vi "Get Shutdown Data.vi"(8 "error in (no error)":errorcluster, 10 "Splitter":refnum<vi>, 11 "Message Log in":refnum<class "Message Log.lvclass">) -> (0 "error out":errorcluster, 2 "Data":T1, 3 "Message Log out":refnum<class "Message Log.lvclass">)   [LabVIEW 2017, in "Message Log.lvclass"]
uses:
  Message Log.lvclass
  Config Data.ctl
  <vilib>/Utility/miscctls.llb/LVRectTypeDef.ctl
  C:/Program Files (x86)/National Instruments/LabVIEW 2017/vi.lib/addons/_Workers/Library/Classes/Worker/Worker.lvclass
  Message Log.lvclass/Message Log.ctl
  <vilib>/addons/_Workers/Library/Classes/Worker/Worker.lvclass/Worker.ctl
  <vilib>/Utility/miscctls.llb/LVRowAndColumnTypeDef.ctl
  <vilib>/addons/_Workers/Library/Classes/Worker/Read MainVI Ref DVR.vi
  <vilib>/addons/_Workers/Library/Classes/Worker/Worker.lvclass
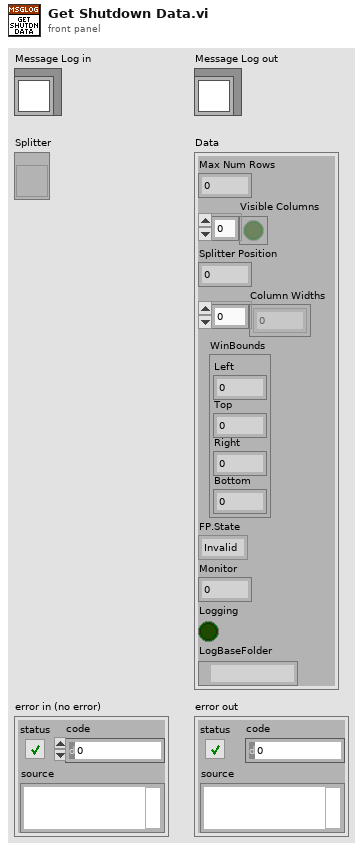
[diagram p1: front panel]
types:
  T1 = typedef "Message Log.lvclass/Config Data.ctl" = cluster{"Max Num Rows":i32, "Visible Columns":bool[], "Splitter Position":i32, "Column Widths":u32[], "WinBounds":T2, "FP.State":enum32{"Invalid", "Standard", "Closed", "Hidden", "Minimized", "Maximized"}, "Monitor":u16, "Logging":bool, "LogBaseFolder":path}
  T2 = typedef "LVRectTypeDef.ctl" = cluster{"Left":i16, "Top":i16, "Right":i16, "Bottom":i16}
  T3 = typedef "LVRowAndColumnTypeDef.ctl" = cluster{"Row":i32, "Column":i32}
  T4 = enum32{"Invalid", "Standard", "Closed", "Hidden", "Minimized", "Maximized"}
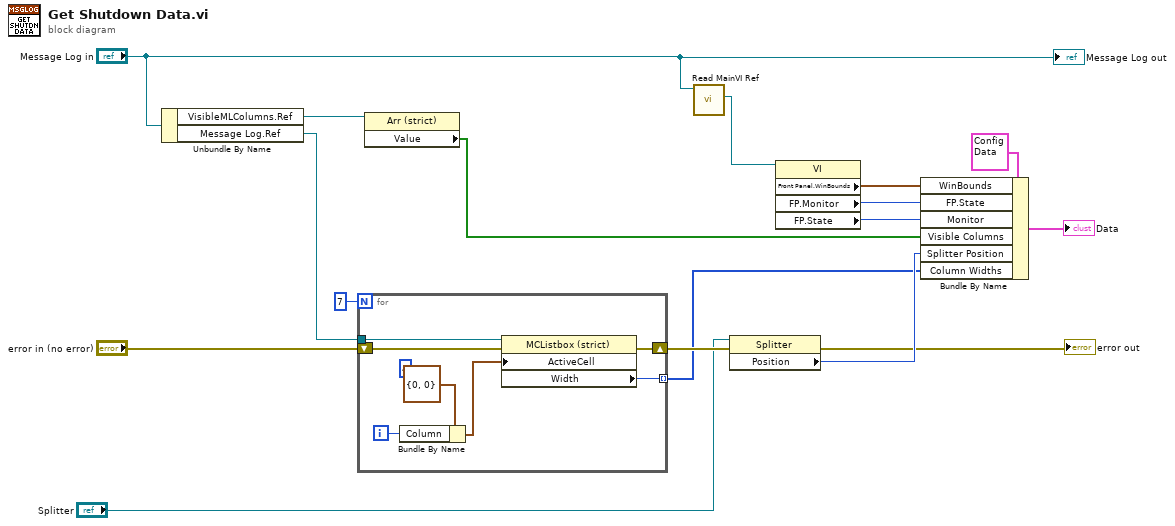
[diagram p0: block diagram]
diagram:
  (unwired) 4
  n1 = Unbundle By Name("Message Log in") -> ("VisibleMLColumns.Ref"=w10:refnum<vi>, "Message Log.Ref"=w7:refnum<vi>)
  n2 = for {
    N: 7 -> [_]
    tunnel: w7 -> [w24]
    shift-right: [w22] -> w13
    shift-left: "error in (no error)" -> [w23]
    tunnel: [w21] -> w9 mode=indexing
    i -> [w19]
    n3 = Bundle By Name(cluster=T3 {"Row"=0, "Column"=0} ("Active Cell:Active Cell"), "Column"=w19) -> (w18:T3)
    n4 = property class="MCListbox (strict)"(reference=w24, error in=w23, "ActiveCell"=w18) -> (error out=w22:errorcluster, "Width"=w21:u32)  [unwired: 1 out]
  }
  n5 = property class="Arr (strict)"(reference=w10) -> ("Value"=w11:bool[])  [unwired: 1 in, 2 out]
  n6 = call <vilib>:"Read MainVI Ref.vi"("Worker_"="Message Log in") -> ("MainVI Ref"=w2:refnum<vi>)  [unwired: 9 in, 1 out]
  n7 = property class="Splitter"(reference="Splitter", error in=w13) -> (error out=→"error out":errorcluster, "Position"=w15:i32)  [unwired: 1 out]
  n8 = property class="VI"(reference=w2) -> ("Front Panel.WinBounds"=w3:T2, "FP.Monitor"=w5:u16, "FP.State"=w4:T4)  [unwired: 1 in, 2 out]
  n9 = Bundle By Name(cluster=T1 {"Max Num Rows"=0, "Visible Columns"=[], "Splitter Position"=0, "Column Widths"=[], "WinBounds"={"Left"=0, "Top"=0, "Right"=0, "Bottom"=0}, "FP.State"=enum."Invalid", "Monitor"=0, "Logging"=FALSE, "LogBaseFolder"=path ""} ("Data"), "WinBounds"=w3, "FP.State"=w4, "Monitor"=w5, "Visible Columns"=w11, "Splitter Position"=w15, "Column Widths"=w9) -> (→"Data":T1)
  "Message Log out" <- "Message Log in"
